vi "Extract Text (static).vi"(7 "Copy":bool caption="Copy data instead of extracting", 8 "error in (no error)":errorcluster, 11 "TextMessage in":refnum<class "MSG.lvclass">) -> (0 "error out":errorcluster, 1 "Text":string, 2 "Label":string, 3 "TextMessage out":refnum<class "MSG.lvclass">)   [LabVIEW 2011, in "Messenging.lvlib" / "MSG.lvclass"]
uses:
  MSG.lvclass
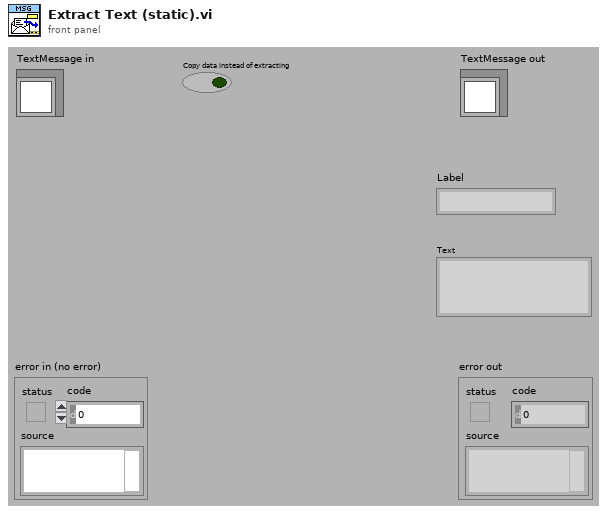
[diagram p1: front panel]
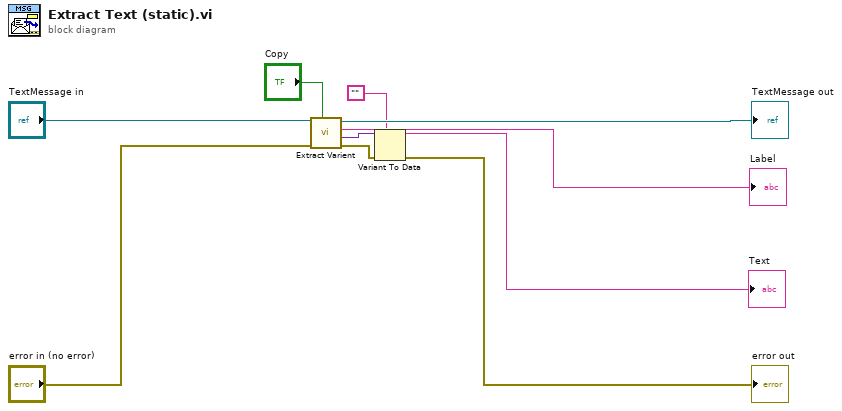
[diagram p0: block diagram]
diagram:
  n1 = call-dynamic "Extract Varient.vi"("Copy"="Copy", "error in (no error)"="error in (no error)", "Message"="TextMessage in") -> ("error out"=w3:errorcluster, "Varient"=w6:variant, "Label"=→"Label":string, "Message"=→"TextMessage out":refnum<class "MSG.lvclass">)  [unwired: 5 out]
  n2 = Variant To Data(error in=w3, type="", Variant=w6) -> (data=→"Text":string, error out=→"error out":errorcluster)
